vi "Calculate-MSCN Dt.vi"(8 "ROI number":i32=1, 9 "[ROI Time(us)]":dbl[](array[numeric]), 11 "Number of pixels in ROI":i32) -> (2 "MSCN Dt":dbl)   [LabVIEW 2017]
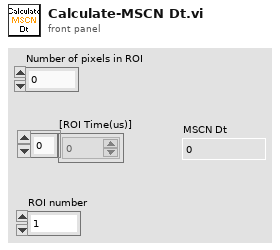
[diagram p1: front panel]
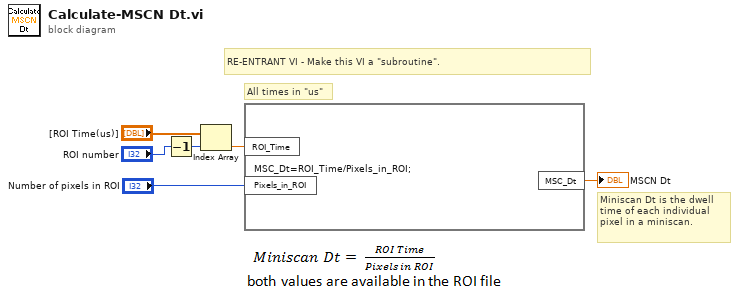
[diagram p0: block diagram]
diagram:
  # "RE-ENTRANT VI - Make this VI a \"subroutine\"."
  # "Miniscan Dt is the dwell time of each individual pixel in a miniscan."
  # "All times in \"us\""
  n1 = Decrement(x="ROI number") -> (x-1=w1:i32)
  n2 = Index Array(array="[ROI Time(us)]", index=w1) -> (element=w3:dbl)
  n3 = formula code="MSC_Dt=ROI_Time/Pixels_in_ROI;"("ROI_Time"=w3, "Pixels_in_ROI"="Number of pixels in ROI") -> ("MSC_Dt"=→"MSCN Dt":dbl)
